vi "Sweep Step.vi"(8 "error in (no error)":errorcluster, 11 "Power Supply in":refnum<class "Power Supply.lvclass">) -> (0 "error out":errorcluster, 1 "Done?":bool, 2 "field":dbl[unit], 3 "Power Supply out":refnum<class "Power Supply.lvclass">, 4 "rate":dbl[unit])   [LabVIEW 2009, in "Power Supply.lvclass"]
doc: "As the field sweeps, monitor that the current sweep rate is still appropriate and adjust as necessary."
uses:
  Power Supply.lvclass
  Ramping Mode.ctl
  Power Supply.lvclass/Power Supply.ctl
panel:
  in  "Ramping Mode":T1
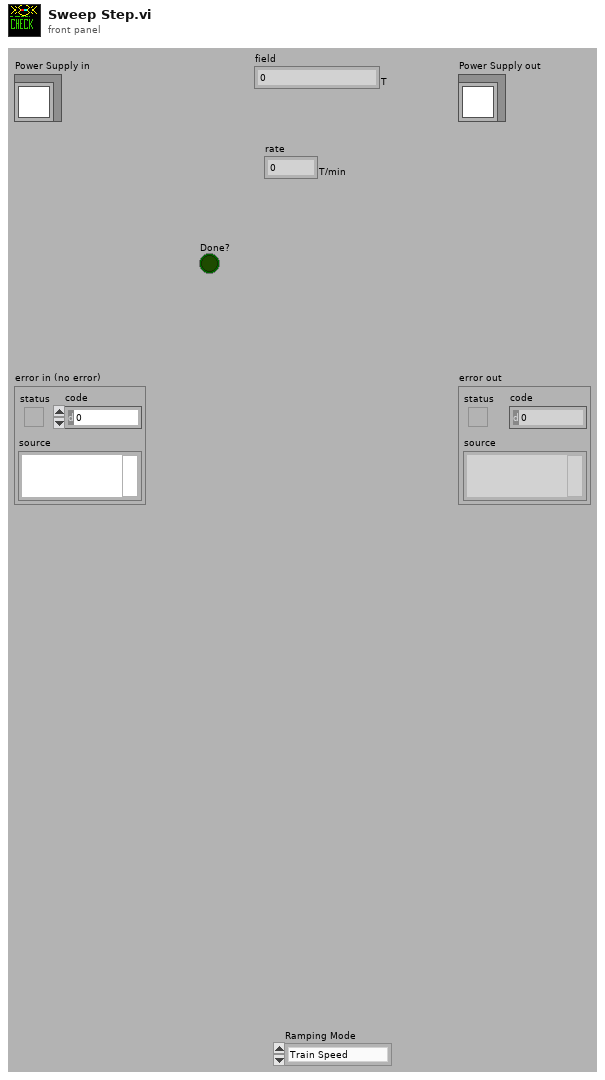
[diagram p1: front panel]
types:
  T1 = typedef "Power Supply.lvclass/Ramping Mode.ctl" = enum16{"Train Speed", "Maximum Speed", "Manual"}
  T2 = typedef "PSIO.ctl" = cluster{"Address":T3, "Version":enum16{"PS", "IPS"}}
  T3 = typedef "OxfordAddress.ctl" = cluster{"Com Port":i32, "ISOBUS Address":i32, "GPIB Address":i16, "Communication":enum16{"RS232", "ISOBUS", "GPIB", "Gateway"}}
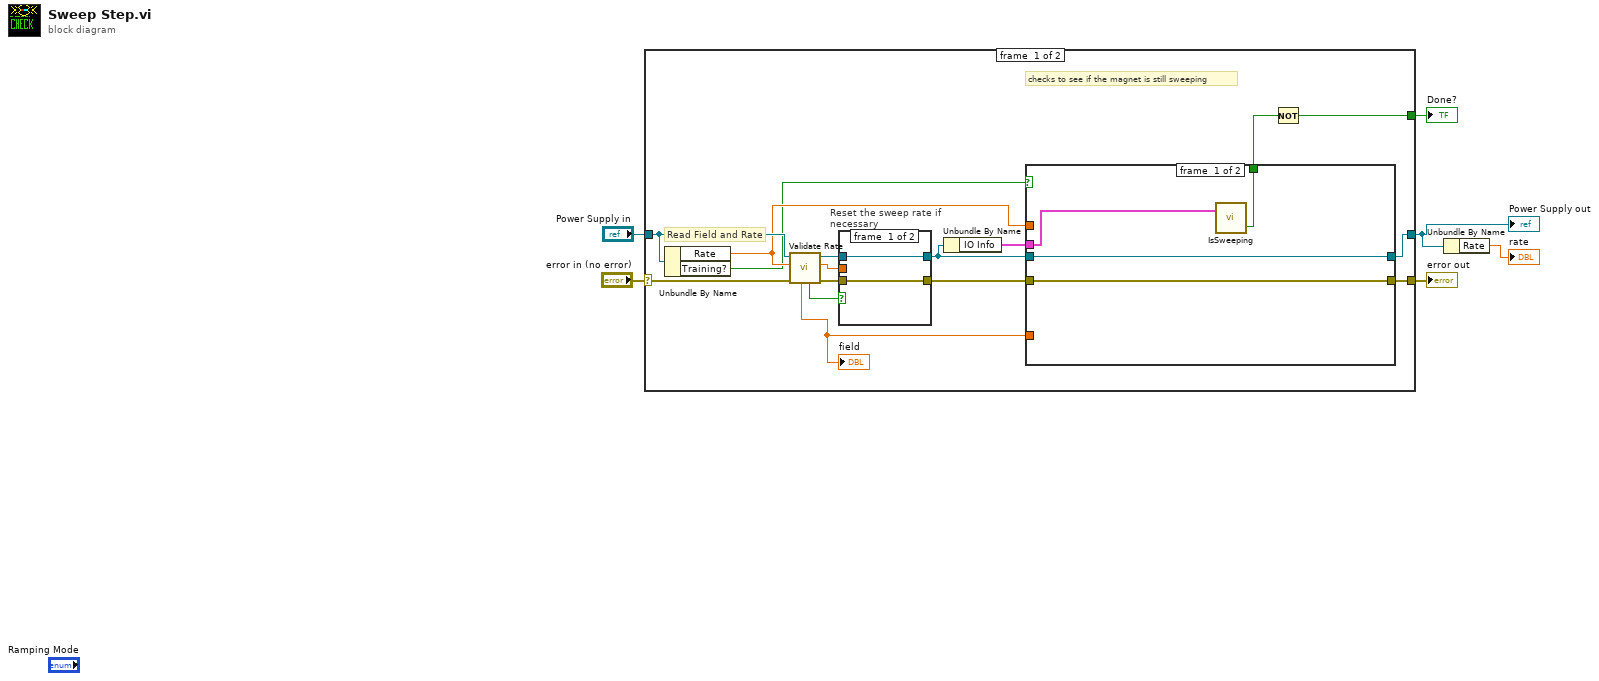
[diagram p0: block diagram]
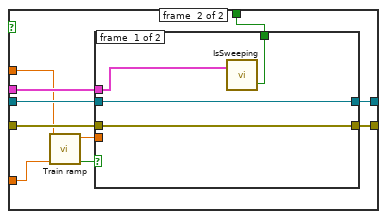
[diagram p2: hidden frame]
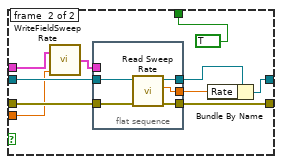
[diagram p3: hidden frame]
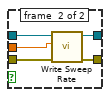
[diagram p4: hidden frame]
diagram:
  n1 = case shown="No Error" "error in (no error)" {
    selector: "error in (no error)" -> [w19 w63]
    tunnel: [w18 _] -> w6
    tunnel: [w16 w63] -> w5
    tunnel: [w12 w64] -> w2
    tunnel: "Power Supply in" -> [w20 w64]
    frame #0 {
      # "checks to see if the magnet is still sweeping"
      # "Read Field and Rate"
      n2 = Unbundle By Name(w20) -> ("Rate"=w9:dbl[unit], "Training?"=w8:bool)
      n3 = call "Validate Rate.vi"("error IO"=w19, "rate"=w9, "Power Supply in"=w20) -> ("error out"=w22:errorcluster, "Coerced rate"=w14:dbl[unit], "Power Supply out"=w21:refnum<class "Power Supply.lvclass">, "Coerced?"=w11:bool, "Field"=w10:dbl[unit])  [unwired: 3 in, 1 out]
      "field" <- w10
      n4 = case "Reset the sweep rate if necessary" shown="True" w11 {
        tunnel: w14 -> [_ w60]
        tunnel: w22 -> [w56 w62]
        tunnel: [w56 w61] -> w17
        tunnel: w21 -> [w57 w59]
        tunnel: [w57 w58] -> w13
        frame #0 {
        }
        frame #1 {
          n5 = call-dynamic "Write Sweep Rate.vi"("error in (no error)"=w62, "rate"=w60, "Power Supply in"=w59) -> ("error out"=w61:errorcluster, "Power Supply out"=w58:refnum<class "Power Supply.lvclass">)  [unwired: 7 in]
        }
      }
      n6 = Unbundle By Name(w13) -> ("IO Info"=w15:T2)
      n7 = case shown="True" w8 {
        tunnel: w17 -> [w25 w36]
        tunnel: [w25 w35] -> w16
        tunnel: w15 -> [w24 w32]
        tunnel: w13 -> [w26 w34]
        tunnel: [w26 w33] -> w12
        tunnel: w10 -> [_ w29]
        tunnel: w9 -> [_ w28]
        tunnel: [w23 w27] -> w7
        frame #0 {
          n8 = call "IsSweeping.vi"("IO Info"=w24) -> ("Sweeping"=w23:bool)  [unwired: 2 out]
        }
        frame #1 {
          n9 = call "Train ramp.vi"("Field"=w29, "Input"=w28) -> ("Change?"=w31:bool, "Output"=w30:dbl[unit])  [unwired: 8 in]
          n10 = case shown="True" w31 {
            tunnel: w36 -> [w39 w48]
            tunnel: [w39 w47] -> w35
            tunnel: w34 -> [w40 w46]
            tunnel: [w40 w45] -> w33
            tunnel: w32 -> [w38 w44]
            tunnel: w30 -> [_ w42]
            tunnel: [w37 TRUE] -> w27
            frame #0 {
              n11 = call "IsSweeping.vi"("IO Info"=w38) -> ("Sweeping"=w37:bool)  [unwired: 2 out]
            }
            frame #1 {
              n12 = call "WriteFieldSweepRate.vi"("Sweep rate"=w42, "IO Info"=w44) -> ("IO Info"=w49:T2)
              n13 = flat-sequence {
                tunnel: [w55] -> w43
                tunnel: w46 -> [w54]
                tunnel: [w53] -> w50
                tunnel: w49 -> [_]
                tunnel: w48 -> [w52]
                tunnel: [w51] -> w47
                frame #0 {
                  n14 = call-dynamic "Read Sweep Rate.vi"("error in (no error)"=w52, "Power Supply in"=w54) -> ("error out"=w51:errorcluster, "Field sweep rate"=w55:dbl[unit], "Power Supply out"=w53:refnum<class "Power Supply.lvclass">)  [unwired: 7 in]
                }
              }
              n15 = Bundle By Name(cluster=w50, "Rate"=w43) -> (w45:refnum<class "Power Supply.lvclass">)
            }
          }
        }
      }
      n16 = Not(x=w7) -> (.not. x?=w18:bool)
    }
    frame #1 {
    }
  }
  "Done?" <- w6
  "error out" <- w5
  "Power Supply out" <- w2
  n17 = Unbundle By Name(w2) -> ("Rate"=→"rate":dbl[unit])
